vi "Children Allowed.vi"(8 "error in (no error)":errorcluster, 11 "BetterTreeItem in":refnum<class "BetterItem.lvclass">) -> (0 "error out":errorcluster, 2 "Child allowed?":bool, 3 "BetterTreeItem out":refnum<class "BetterItem.lvclass">)   [LabVIEW 2020, in "BetterDragAndDrop.lvlib" / "BetterItem.lvclass"]
uses:
  BetterItem.lvclass
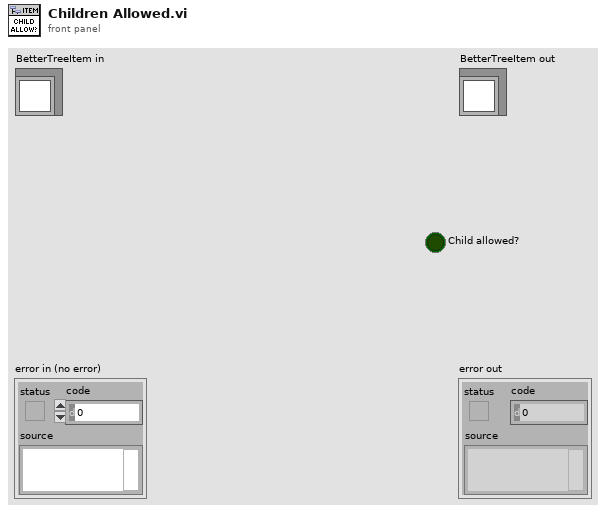
[diagram p1: front panel]
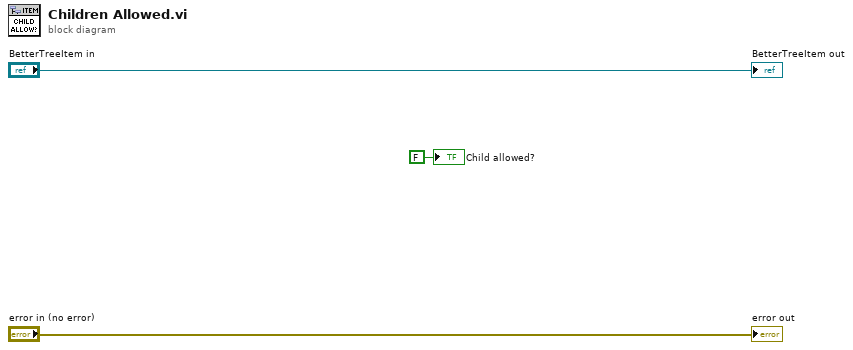
[diagram p0: block diagram]
diagram:
  "error out" <- "error in (no error)"
  "BetterTreeItem out" <- "BetterTreeItem in"
  "Child allowed?" <- FALSE ("Child allowed?")
